vi "add_multiple_scales_to_graph.vi"() -> ()   [LabVIEW 2013]
panel:
  in  "stop":bool
  in  "Show Axis 4":bool
  in  "Show Axis 3":bool
  in  "Show Axis 2":bool
  in  "Show Axis 1":bool=TRUE
  out "Waveform Graph":dbl[](graph)
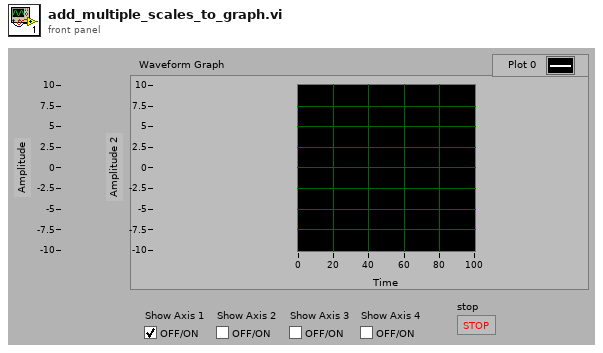
[diagram p1: front panel]
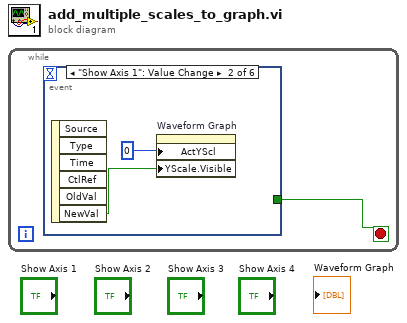
[diagram p0: block diagram]
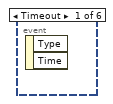
[diagram p2: hidden frame]
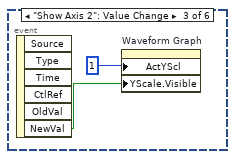
[diagram p3: hidden frame]
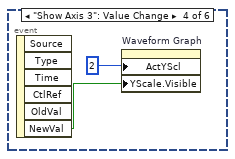
[diagram p4: hidden frame]
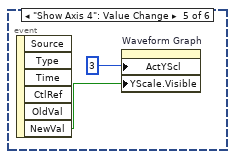
[diagram p5: hidden frame]
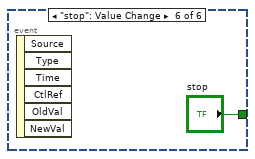
[diagram p6: hidden frame]
diagram:
  n1 = while {
    stop <- w1 stop-if-true
    n2 = event shown="[1] \"Show Axis 1\": Value Change" {
      selector: _ -> [_ _ _ _ _ _]
      dyn-events: _ -> [_ _ _ _ _ _]
      timeout: _ -> [_ _ _ _ _ _]
      tunnel: [_ _ _ _ _ "stop"] -> w1
      event Timeout {
        n3 = event-data() -> ()  [unwired: 1 in, 2 out]
      }
      event "Show Axis 1": Value Change {
        n4 = event-data() -> ("NewVal"=w2:bool)  [unwired: 1 in, 5 out]
        n5 = property on="Waveform Graph" class="WFGraph (strict)"("ActYScl"=0 ("Active Y Scale"), "YScale.Visible"=w2) -> ()  [unwired: 2 in, 2 out]
      }
      event "Show Axis 2": Value Change {
        n6 = event-data() -> ("NewVal"=w4:bool)  [unwired: 1 in, 5 out]
        n7 = property on="Waveform Graph" class="WFGraph (strict)"("ActYScl"=1 ("Active Y Scale"), "YScale.Visible"=w4) -> ()  [unwired: 2 in, 2 out]
      }
      event "Show Axis 3": Value Change {
        n8 = event-data() -> ("NewVal"=w6:bool)  [unwired: 1 in, 5 out]
        n9 = property on="Waveform Graph" class="WFGraph (strict)"("ActYScl"=2 ("Active Y Scale"), "YScale.Visible"=w6) -> ()  [unwired: 2 in, 2 out]
      }
      event "Show Axis 4": Value Change {
        n10 = event-data() -> ("NewVal"=w8:bool)  [unwired: 1 in, 5 out]
        n11 = property on="Waveform Graph" class="WFGraph (strict)"("ActYScl"=3 ("Active Y Scale"), "YScale.Visible"=w8) -> ()  [unwired: 2 in, 2 out]
      }
      event "stop": Value Change {
        n12 = event-data() -> ()  [unwired: 1 in, 6 out]
      }
    }
  }
